vi "Batch Detect.vi"(7 "Unit ID (A)":string="A", 8 "error in":errorcluster, 11 "VISA Session In":refnum<visa-resource-name>="Alicat") -> (0 "error out":errorcluster, 2 "Batching available":bool, 3 "VISA Session Out":refnum<visa-resource-name>)   [LabVIEW 2014]
doc: "Checks whether the Alicat device supports batch setpoints or not."
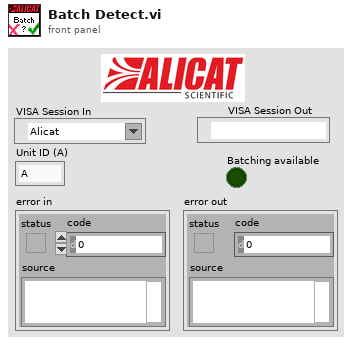
[diagram p1: front panel]
types:
  T1 = enum8{"No Totalizer", "Mass Flow", "Volumetric Flow"}
  T2 = cluster{"Controller Select":u16, "SetPoint Source":enum8{"Serial", "Local", "Analog", "Unknown"}, "AutoTare":enum16{"Disabled", "Enabled"}}
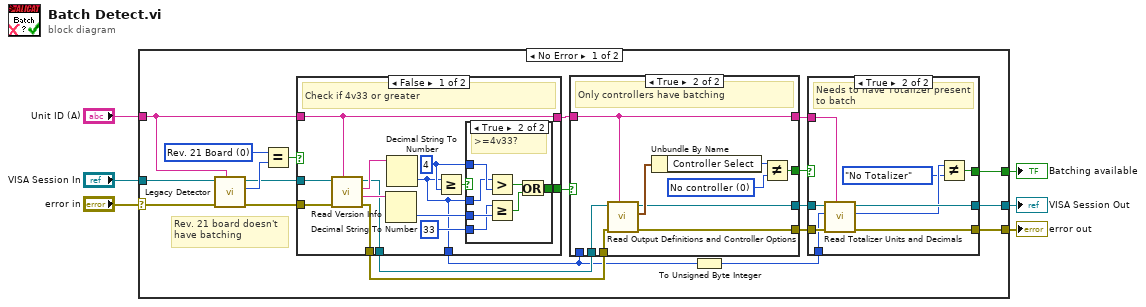
[diagram p0: block diagram]
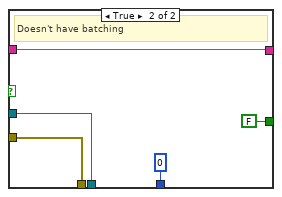
[diagram p5: hidden frame]
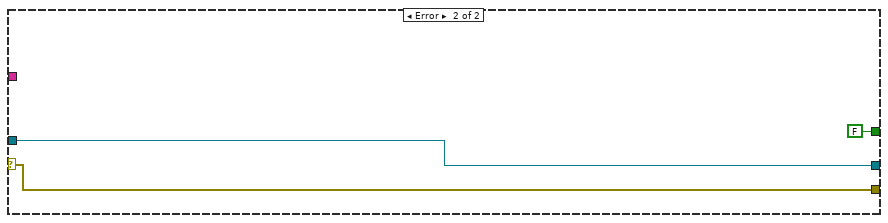
[diagram p6: hidden frame]
diagram:
  n1 = case shown="No Error" "error in" {
    selector: "error in" -> [w9 w80]
    tunnel: "VISA Session In" -> [w27 w81]
    tunnel: "Unit ID (A)" -> [w24 _]
    tunnel: [w12 FALSE] -> w4
    tunnel: [w11 w81] -> w3
    tunnel: [w10 w80] -> w2
    frame No Error {
      w26 = u8 0 items=["Rev. 21 Board", "Rev. 22 Board", "Rev. 23 Board"] ("Legacy Status")
      # "Rev. 21 board doesn't\nhave batching"
      n2 = call "Legacy Detector.vi"("Unit ID (A)"=w24, "error in"=w9, "VISA Session In"=w27) -> ("error out"=w21:errorcluster, "Legacy Status"=w25:u8, "VISA Session Out"=w23:refnum<visa-resource-name>)  [unwired: 6 in]
      n3 = Equal?(x=w26, y=w25) -> (x = y?=w22:bool)
      n4 = case shown="False" w22 {
        tunnel: w24 -> [w54 w77]
        tunnel: w23 -> [w65 w76]
        tunnel: w21 -> [w64 w75]
        tunnel: [w57 FALSE] -> w20
        tunnel: [w56 w76] -> w18
        tunnel: [w55 w75] -> w19
        tunnel: [w54 w77] -> w17
        tunnel: [w53 0] -> w8
        frame False {
          w59 = 4 ("y")
          # "Check if 4v33 or greater"
          n5 = call "Read Version Info.vi"("Unit ID (A)"=w54, "error in"=w64, "VISA Session In"=w65) -> ("error out"=w55:errorcluster, "Software Sub-Rev"=w62:string, "Software Rev"=w63:string, "VISA Session Out"=w56:refnum<visa-resource-name>)  [unwired: 4 in, 1 out]
          n6 = Decimal String To Number(string=w62) -> (number=w60:i32)  [unwired: 2 in, 1 out]
          n7 = Decimal String To Number(string=w63) -> (number=w53:i32)  [unwired: 2 in, 1 out]
          n8 = Greater Or Equal?(x=w53, y=w59) -> (x >= y?=w61:bool)
          n9 = case shown="True" w61 {
            selector: w61 -> [w66 _]
            tunnel: w60 -> [_ w70]
            tunnel: w53 -> [_ w72]
            tunnel: w59 -> [_ w73]
            tunnel: 33 ("y") -> [_ w69]
            tunnel: [w66 w67] -> w57
            frame False {
            }
            frame True {
              # ">=4v33?"
              n10 = Greater?(x=w72, y=w73) -> (0:w71:bool)
              n11 = Greater Or Equal?(x=w69, y=w70) -> (x >= y?=w68:bool)
              n12 = Or(x=w71, y=w68) -> (x .or. y?=w67:bool)
            }
          }
        }
        frame True {
          # "Doesn't have batching"
        }
      }
      n13 = case shown="True" w20 {
        selector: w20 -> [w41 _]
        tunnel: w19 -> [w42 w50]
        tunnel: w18 -> [w43 w49]
        tunnel: [w42 w48] -> w14
        tunnel: [w43 w47] -> w15
        tunnel: w17 -> [w40 w45]
        tunnel: [w41 w46] -> w16
        tunnel: [w40 w45] -> w13
        tunnel: w8 -> [_ _]
        frame False {
          # "Already failed previous check"
        }
        frame True {
          w44 = u16 0 items=["No controller"=0, "Volumetric Flow"=36, "Mass Flow"=37, "Absolute Pressure"=34, "Gauge Pressure"=38, "Differential Pressure"=39] ("Controller Select")
          # "Only controllers have batching"
          n14 = call "Read Output Definitions and Controller Options.vi"("Unit ID (A)"=w45, "error in"=w50, "VISA Session In"=w49) -> ("error out"=w48:errorcluster, "Read/Write Options"=w52:T2, "VISA Session Out"=w47:refnum<visa-resource-name>)  [unwired: 5 in, 1 out]
          n15 = Unbundle By Name(w52) -> ("Controller Select"=w51:u16)
          n16 = Not Equal?(x=w51, y=w44) -> (x != y?=w46:bool)
        }
      }
      n17 = To Unsigned Byte Integer(number=w8) -> (unsigned 8bit integer=w7:u8)
      n18 = case shown="True" w16 {
        selector: w16 -> [w30 _]
        tunnel: w13 -> [_ w37]
        tunnel: w15 -> [w29 w39]
        tunnel: w14 -> [w28 w38]
        tunnel: [w29 w36] -> w11
        tunnel: [w28 w35] -> w10
        tunnel: [w30 w32] -> w12
        tunnel: w7 -> [_ w31]
        frame False {
          # "Already failed previous check"
        }
        frame True {
          # "Needs to have Totalizer present to batch"
          n19 = call "Read Totalizer Units and Decimals.vi"("Unit ID (A)"=w37, "error in"=w38, "Software Version"=w31, "VISA Session In"=w39) -> ("error out"=w35:errorcluster, "Totalizer"=w34:T1, "VISA Session Out"=w36:refnum<visa-resource-name>)  [unwired: 3 in, 2 out]
          n20 = Not Equal?(x=w34, y=T1."No Totalizer") -> (x != y?=w32:bool)
        }
      }
    }
    frame Error {
    }
  }
  "error out" <- w2
  "VISA Session Out" <- w3
  "Batching available" <- w4
